vi "TrigonometricFunctions.vi"(7 "摆角采样":dbl, 8 "力采样N":dbl) -> (5 "力矩采样Nm":dbl, 6 "力臂":dbl)   [LabVIEW 2020]
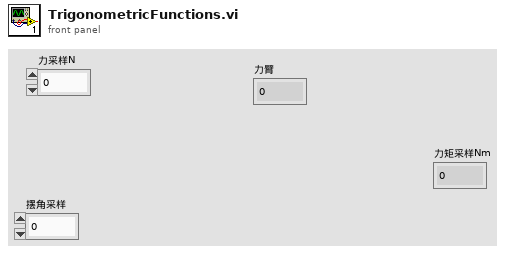
[diagram p1: front panel]
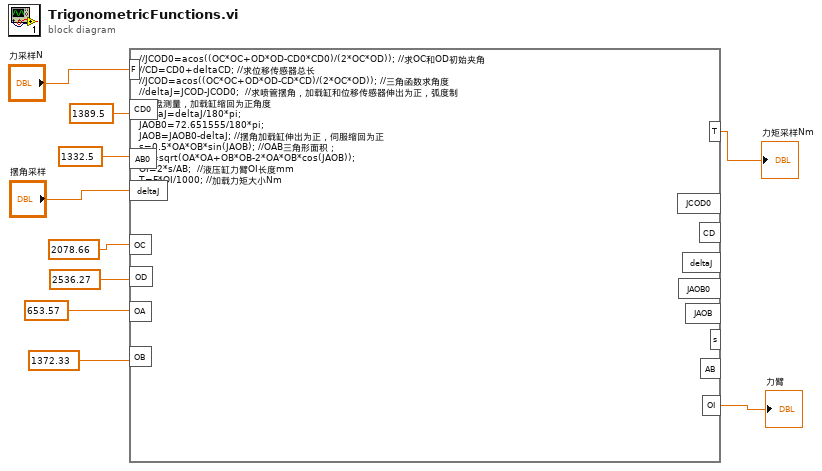
[diagram p0: block diagram]
diagram:
  n1 = formula code="//JCOD0=acos((OC*OC+OD*OD-CD0*CD0)/(2*OC*OD)); //求OC和OD初始夹角\n//CD=CD0+deltaCD; //求位移传感器总长\n//JCOD=acos((OC*OC+OD*OD-CD*CD)/(2*OC*OD)); //三角函数求角度\n//deltaJ=JCOD-JCOD0;  //求喷管摆角，加载缸和位移传感器伸出为正，弧度制\n//码盘测量，加载缸缩回为正角度\ndeltaJ=deltaJ/180*pi;\nJAOB0=72.651555/180*pi;\nJAOB=JAOB0-deltaJ; //摆角加载缸伸出为正，伺服缩回为正\ns=0.5*OA*OB*sin(JAOB); //OAB三角形面积；\nAB=sqrt(OA*OA+OB*OB-2*OA*OB*cos(JAOB));\nOI=2*s/AB;  //液压缸力臂OI长度mm\nT=F*OI/1000; //加载力矩大小Nm"("CD0"=1389.5, "AB0"=1332.5, "deltaJ"="摆角采样", "F"="力采样N", "OC"=2078.66, "OD"=2536.27, "OA"=653.57, "OB"=1372.33) -> ("T"=→"力矩采样Nm":dbl, "OI"=→"力臂":dbl)  [unwired: 7 out]
